vi "SiosIfmGetRecentValues.vi"(1 "index":i32, 2 "int32DeviceNumber":i32) -> (0 "success":bool)   [LabVIEW 2009]
uses:
  siosifm.dll
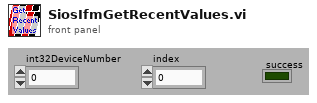
[diagram p1: front panel]
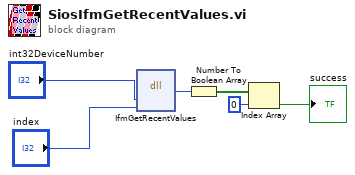
[diagram p0: block diagram]
diagram:
  n1 = dll-call lib="D:/Support/Labview/RE-10/SIOS_IfmDLL/siosifm.dll" fn="IfmGetRecentValues"("deviceNumber"="int32DeviceNumber", "index"="index") -> ("success"=w1:i32)  [unwired: 5 in, 2 out]
  n2 = Number To Boolean Array(number=w1) -> (Boolean array=w3:bool[])
  n3 = Index Array(array=w3, index=0 ("Index")) -> (element=→"success":bool)
